vi "探头窗口-28-4列.vi"() -> ()   [LabVIEW 2017]
panel:
  in  "更新数据":T1
  in  "停止信号":bool=TRUE
  out "更新数据？":bool=TRUE
  out "引用-切回列表模式？":refnum<vi>
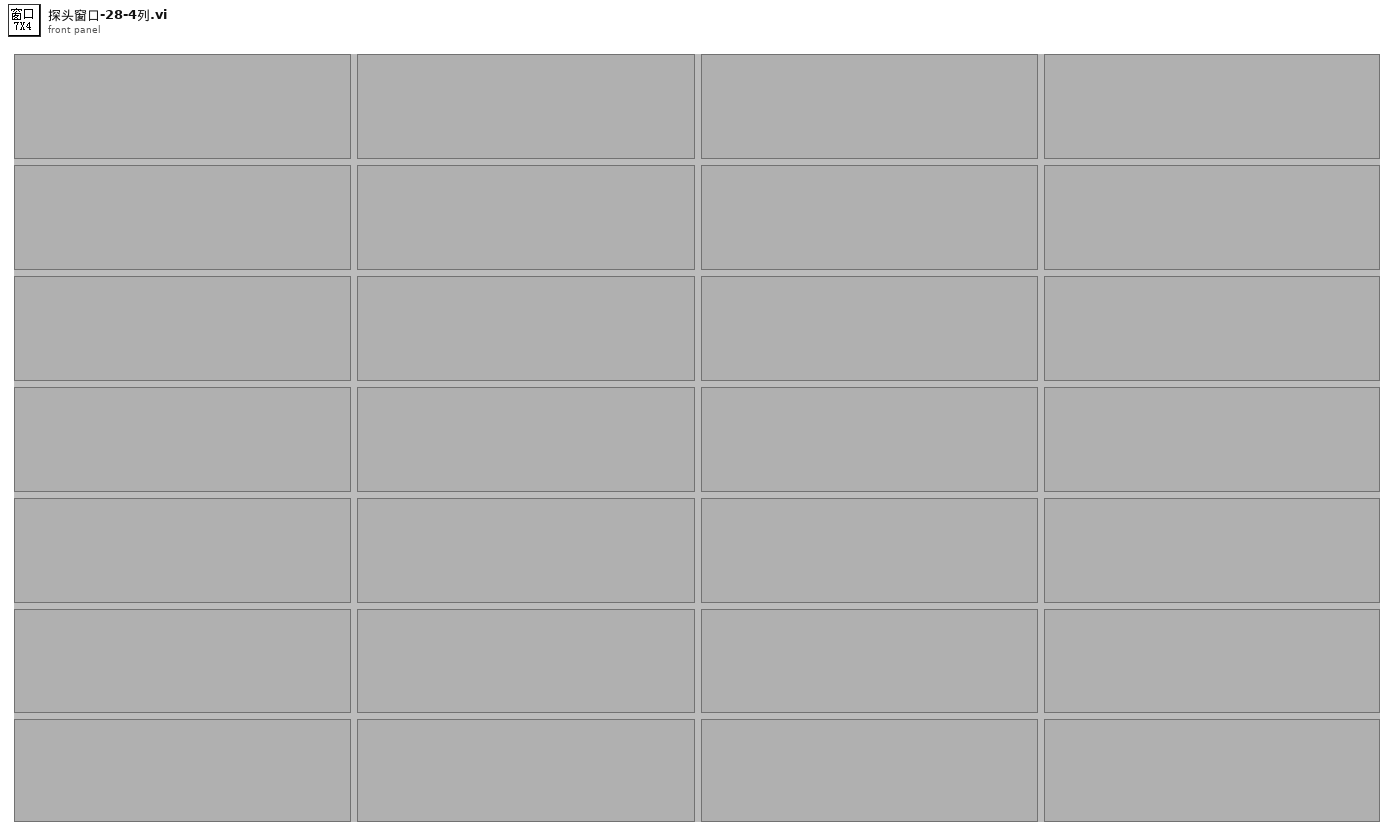
[diagram p1: front panel]
types:
  T1 = cluster{"探头启用状态？":bool[], "测量值":cluster{"X":timestamp, "Y":dbl}[], "限值":cluster{"限值1":dbl, "限值2":dbl, "探头限值":enum16{"一级限值", "二级限值"}}[], "报警状态":enum16{"正常", "一级报警", "二级报警", "累积报警"}[], "探头信息":string[], "累积剂量":cluster{"设备名称":string, "启用累积？":bool, "起始时间":timestamp, "累积剂量":dbl, "累积报警阈值":dbl}[]}
  T2 = cluster{"启用状态？":bool, "测量值":cluster{"X":timestamp, "Y":dbl}, "限值簇":cluster{"限值1":dbl, "限值2":dbl, "探头限值":enum16{"一级限值", "二级限值"}}, "报警状态":enum16{"正常", "一级报警", "二级报警", "累积报警"}, "探头信息":string, "探头地址":i32, "累积剂量":cluster{"设备名称":string, "启用累积？":bool, "起始时间":timestamp, "累积剂量":dbl, "累积报警阈值":dbl}}
  T3 = typedef "eventvkey.ctl" = enum16{"ASCII", "Enter", "Return", "Shift", "Ctrl", "Alt", "Cmd", "Opt", "Caps", "NumLock", "Clear", "Break", "Up", "Down", "Left", "Right", "Insert", "Delete", "Home", "End", "PageUp", "PageDown", "Escape", "Help", "Pause", "ScrollLock", "F1", "F2", "F3", "F4", "F5", "F6", "F7", "F8", "F9", "F10", "F11", "F12", "F13", "F14", "F15", "F16", "F17", "F18", "F19", "F20", "F21", "F22", "F23", "F24", "Play", "VolumeUp", "VolumeDown", "Mute", "Two Byte Char"}
  T4 = cluster{"限值1":dbl, "限值2":dbl, "探头限值":enum16{"一级限值", "二级限值"}}
  T5 = cluster{"限值1":dbl, "限值2":dbl, "探头限值":enum16{"一级限值", "二级限值"}}[]
  T6 = cluster{"设备名称":string, "启用累积？":bool, "起始时间":timestamp, "累积剂量":dbl, "累积报警阈值":dbl}[]
  T7 = cluster{"设备名称":string, "启用累积？":bool, "起始时间":timestamp, "累积剂量":dbl, "累积报警阈值":dbl}
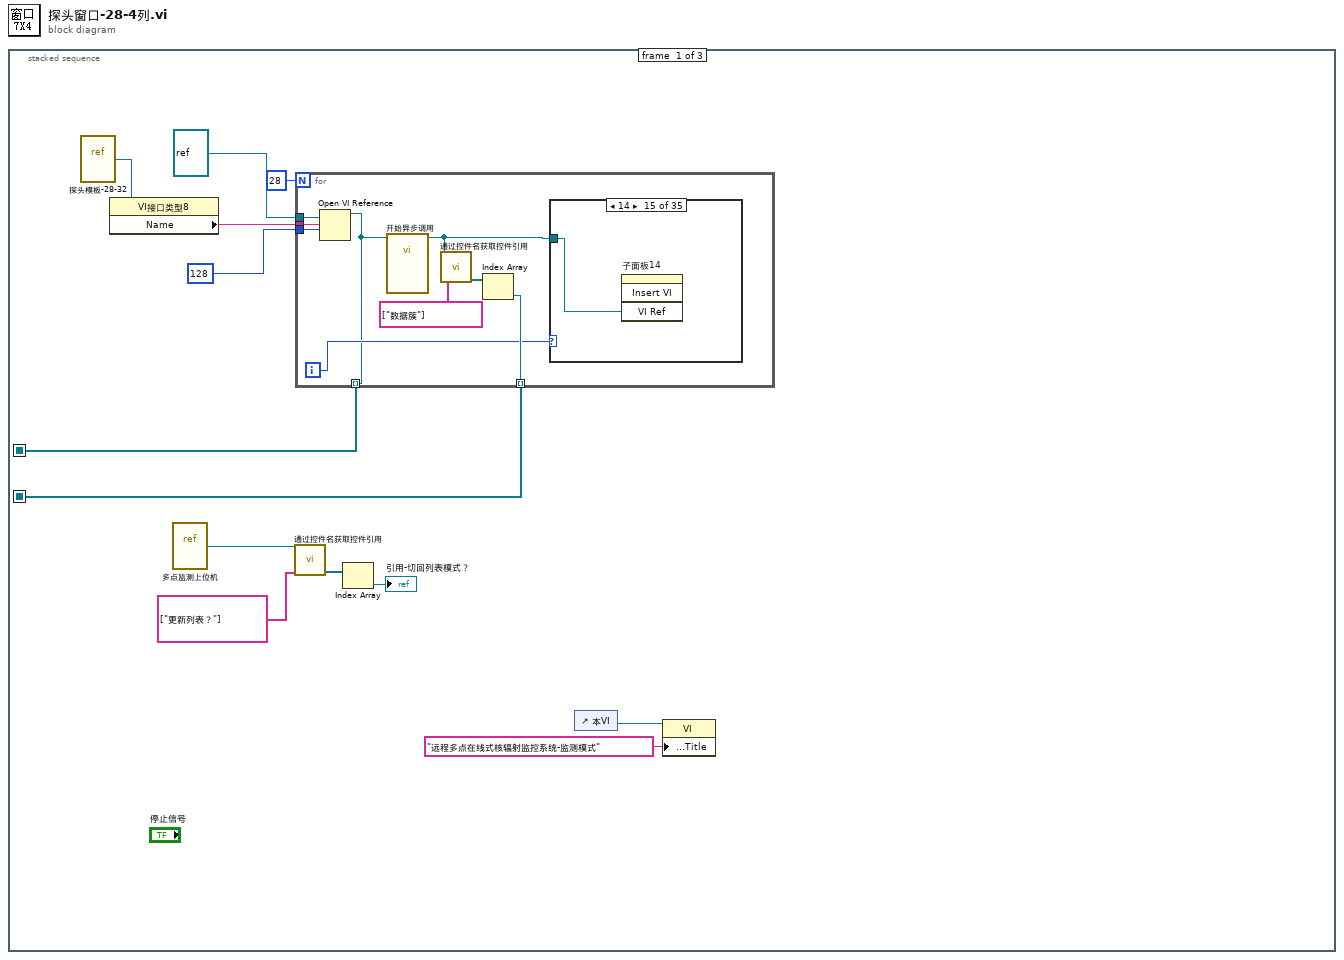
[diagram p0: block diagram]
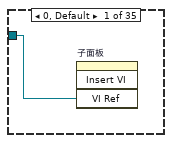
[diagram p2: hidden frame]
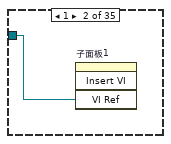
[diagram p3: hidden frame]
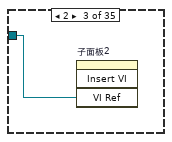
[diagram p4: hidden frame]
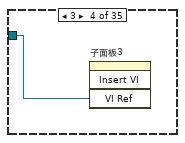
[diagram p5: hidden frame]
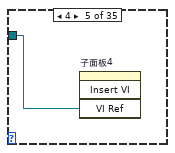
[diagram p6: hidden frame]
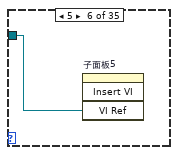
[diagram p7: hidden frame]
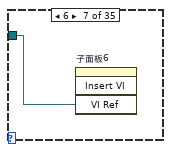
[diagram p8: hidden frame]
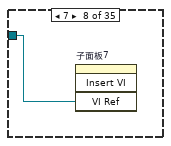
[diagram p9: hidden frame]
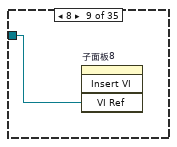
[diagram p10: hidden frame]
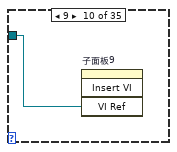
[diagram p11: hidden frame]
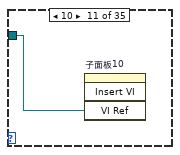
[diagram p12: hidden frame]
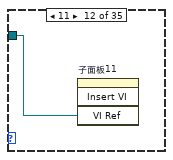
[diagram p13: hidden frame]
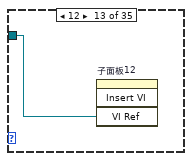
[diagram p14: hidden frame]
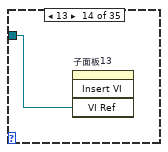
[diagram p15: hidden frame]
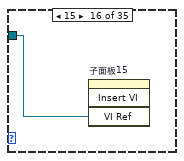
[diagram p16: hidden frame]
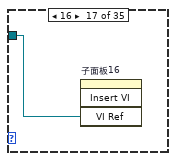
[diagram p17: hidden frame]
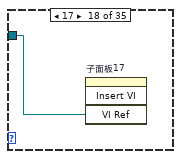
[diagram p18: hidden frame]
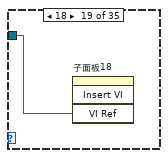
[diagram p19: hidden frame]
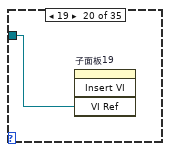
[diagram p20: hidden frame]
diagram:
  n1 = stacked-sequence {
    seq-local: [w8 _ _] -> [_ w52 _]
    seq-local: [w3 _ _] -> [_ w51 _]
    frame #0 {
      n2 = vi-ref "探头模板-28-32.vi"() -> (w13:refnum<vi>)
      n3 = property class="VI接口类型8"(reference=w13) -> ("Name"=w12:string)  [unwired: 1 in, 2 out]
      n4 = vi-ref "多点监测上位机.vi"() -> (w4:refnum<vi>)
      n5 = call "通过控件名获取控件引用.vi"("控件名数组"=string[] ["更新列表？"], "VI引用"=w4) -> ("控件引用输出"=w6:refnum<vi>[])  [unwired: 7 in, 2 out]
      n6 = for {
        N: 28 -> [_]
        tunnel: w12 -> [w22]
        tunnel: 128 ("选项") -> [w21]
        tunnel: refnum<vi> refnum ("类型说明符VI引用句柄（仅用于类型）") -> [w20]
        tunnel: [w15] -> w8 mode=indexing
        tunnel: [w17] -> w3 mode=indexing
        i -> [w16]
        n7 = Open VI Reference(type specifier VI Refnum (for type only)=w20, vi path=w22, options=w21) -> (vi reference=w15:refnum<vi>)  [unwired: 3 in, 1 out]
        n8 = call-by-ref "开始异步调用"(reference=w15) -> (reference out=w14:refnum<vi>)  [unwired: 13 in, 1 out]
        n9 = call "通过控件名获取控件引用.vi"("控件名数组"=string[] ["数据簇"], "VI引用"=w14) -> ("控件引用输出"=w19:refnum<vi>[])  [unwired: 7 in, 2 out]
        n10 = Index Array(array=w19) -> (element=w17:refnum<vi>)  [unwired: 1 in]
        n11 = case shown="14" w16 {
          tunnel: w14 -> [w23 w24 w25 w26 w27 w28 w29 w30 w31 w32 w33 w34 w35 w36 w37 w38 w39 w40 w41 w42 w43 w44 w45 w46 w47 w48 w49 w50 _ _ _ _ _ _ _]
          frame 0, Default {
            n12 = invoke on="子面板" class="子面板" method="Insert VI"("VI Ref"=w23) -> ()  [unwired: 3 in, 4 out]
          }
          frame 1 {
            n13 = invoke on="子面板1" class="SubPnl" method="Insert VI"("VI Ref"=w24) -> ()  [unwired: 3 in, 4 out]
          }
          frame 2 {
            n14 = invoke on="子面板2" class="SubPnl" method="Insert VI"("VI Ref"=w25) -> ()  [unwired: 3 in, 4 out]
          }
          frame 3 {
            n15 = invoke on="子面板3" class="SubPnl" method="Insert VI"("VI Ref"=w26) -> ()  [unwired: 3 in, 4 out]
          }
          frame 4 {
            n16 = invoke on="子面板4" class="SubPnl" method="Insert VI"("VI Ref"=w27) -> ()  [unwired: 3 in, 4 out]
          }
          frame 5 {
            n17 = invoke on="子面板5" class="SubPnl" method="Insert VI"("VI Ref"=w28) -> ()  [unwired: 3 in, 4 out]
          }
          frame 6 {
            n18 = invoke on="子面板6" class="SubPnl" method="Insert VI"("VI Ref"=w29) -> ()  [unwired: 3 in, 4 out]
          }
          frame 7 {
            n19 = invoke on="子面板7" class="SubPnl" method="Insert VI"("VI Ref"=w30) -> ()  [unwired: 3 in, 4 out]
          }
          frame 8 {
            n20 = invoke on="子面板8" class="SubPnl" method="Insert VI"("VI Ref"=w31) -> ()  [unwired: 3 in, 4 out]
          }
          frame 9 {
            n21 = invoke on="子面板9" class="SubPnl" method="Insert VI"("VI Ref"=w32) -> ()  [unwired: 3 in, 4 out]
          }
          frame 10 {
            n22 = invoke on="子面板10" class="SubPnl" method="Insert VI"("VI Ref"=w33) -> ()  [unwired: 3 in, 4 out]
          }
          frame 11 {
            n23 = invoke on="子面板11" class="SubPnl" method="Insert VI"("VI Ref"=w34) -> ()  [unwired: 3 in, 4 out]
          }
          frame 12 {
            n24 = invoke on="子面板12" class="SubPnl" method="Insert VI"("VI Ref"=w35) -> ()  [unwired: 3 in, 4 out]
          }
          frame 13 {
            n25 = invoke on="子面板13" class="SubPnl" method="Insert VI"("VI Ref"=w36) -> ()  [unwired: 3 in, 4 out]
          }
          frame 14 {
            n26 = invoke on="子面板14" class="SubPnl" method="Insert VI"("VI Ref"=w37) -> ()  [unwired: 3 in, 4 out]
          }
          frame 15 {
            n27 = invoke on="子面板15" class="SubPnl" method="Insert VI"("VI Ref"=w38) -> ()  [unwired: 3 in, 4 out]
          }
          frame 16 {
            n28 = invoke on="子面板16" class="SubPnl" method="Insert VI"("VI Ref"=w39) -> ()  [unwired: 3 in, 4 out]
          }
          frame 17 {
            n29 = invoke on="子面板17" class="SubPnl" method="Insert VI"("VI Ref"=w40) -> ()  [unwired: 3 in, 4 out]
          }
          frame 18 {
            n30 = invoke on="子面板18" class="SubPnl" method="Insert VI"("VI Ref"=w41) -> ()  [unwired: 3 in, 4 out]
          }
          frame 19 {
            n31 = invoke on="子面板19" class="SubPnl" method="Insert VI"("VI Ref"=w42) -> ()  [unwired: 3 in, 4 out]
          }
          frame 20 {
            n32 = invoke on="子面板20" class="SubPnl" method="Insert VI"("VI Ref"=w43) -> ()  [unwired: 3 in, 4 out]
          }
          frame 21 {
            n33 = invoke on="子面板21" class="SubPnl" method="Insert VI"("VI Ref"=w44) -> ()  [unwired: 3 in, 4 out]
          }
          frame 22 {
            n34 = invoke on="子面板22" class="SubPnl" method="Insert VI"("VI Ref"=w45) -> ()  [unwired: 3 in, 4 out]
          }
          frame 23 {
            n35 = invoke on="子面板23" class="SubPnl" method="Insert VI"("VI Ref"=w46) -> ()  [unwired: 3 in, 4 out]
          }
          frame 24 {
            n36 = invoke on="子面板24" class="SubPnl" method="Insert VI"("VI Ref"=w47) -> ()  [unwired: 3 in, 4 out]
          }
          frame 25 {
            n37 = invoke on="子面板25" class="SubPnl" method="Insert VI"("VI Ref"=w48) -> ()  [unwired: 3 in, 4 out]
          }
          frame 26 {
            n38 = invoke on="子面板26" class="SubPnl" method="Insert VI"("VI Ref"=w49) -> ()  [unwired: 3 in, 4 out]
          }
          frame 27 {
            n39 = invoke on="子面板27" class="SubPnl" method="Insert VI"("VI Ref"=w50) -> ()  [unwired: 3 in, 4 out]
          }
          frame 28 {
          }
          frame 29 {
          }
          frame 30 {
          }
          frame 31 {
          }
          frame 32 {
          }
          frame 33 {
          }
          frame 34 {
          }
        }
      }
      n40 = Index Array(array=w6) -> (element=→"引用-切回列表模式？":refnum<vi>)  [unwired: 1 in]
      n41 = control-ref of="本VI"() -> (w2:refnum<vi>)
      n42 = property class="VI"(reference=w2, "Front Panel.Title"="远程多点在线式核辐射监控系统-监测模式" ("前面板窗口:标题")) -> ()  [unwired: 1 in, 2 out]
    }
    frame #1 {
      n43 = while {
        tunnel: w52 -> [w54]
        tunnel: w51 -> [w53]
        stop <- w55 stop-if-true
        n44 = event shown="[4] \"更新数据？\": 值改变" {
          selector: _ -> [_ _ _ _ _]
          dyn-events: _ -> [_ _ _ _ _]
          timeout: _ -> [_ _ _ _ _]
          tunnel: [_ TRUE ("放弃？") _ _ _] -> w55
          tunnel: w54 -> [_ w58 _ _ _]
          tunnel: w53 -> [_ _ _ _ w67]
          event Timeout {
            n45 = event-data() -> ()  [unwired: 1 in, 3 out]
          }
          event "停止信号": Value Change {
            w57 = TRUE  # T
            n46 = event-data() -> ()  [unwired: 1 in, 6 out]
            n47 = local read "引用-切回列表模式？"() -> (w56:refnum<vi>)
            n48 = for {
              tunnel: w58 -> [w63] mode=indexing
              n49 = invoke class="VI (严格)" method="Abort VI"(reference=w63) -> (reference out=w61:refnum<vi>, error out=w62:errorcluster)  [unwired: 2 in, 1 out]
              n50 = Close Reference(reference=w61, error in (no error)=w62) -> (error out=w60:errorcluster)
              n51 = call <vilib>:"Clear Errors.vi"("error in (no error)"=w60) -> ()  [unwired: 5 in, 2 out]
            }
            n52 = property class="Ctl"(reference=w56, "Val(Sgnl)"=w57) -> ()  [unwired: 1 in, 2 out]
          }
          event Panel Close? {
            n53 = event-data() -> ()  [unwired: 1 in, 4 out]
            n54 = property on="停止信号" class="Bool (严格)"("Val(Sgnl)"=FALSE ("值(信号)")) -> ()  [unwired: 2 in, 2 out]
            n55 = event-data() -> ()  [unwired: 2 in, 1 out]
          }
          event Key Down {
            n56 = event-data() -> ("VKey"=w65:T3)  [unwired: 1 in, 9 out]
            n57 = case shown="\"Escape\"" w65 {
              frame "ASCII", Default {
              }
              frame "Escape" {
                w66 = TRUE  # T
                n58 = property on="停止信号" class="Bool (严格)"("Val(Sgnl)"=w66) -> ()  [unwired: 2 in, 2 out]
              }
            }
          }
          event "更新数据？": Value Change {
            (unwired) T4 {"限值1"=0.0, "限值2"=0.0, "探头限值"=enum."一级限值"} ("探头限值簇")
            n59 = event-data() -> ()  [unwired: 1 in, 6 out]
            n60 = Unbundle By Name("更新数据") -> ("探头启用状态？"=w68:bool[], "测量值"=w69:cluster{"X":timestamp, "Y":dbl}[], "限值"=w70:T5, "报警状态"=w71:enum16{"正常", "一级报警", "二级报警", "累积报警"}[], "探头信息"=w72:string[], "累积剂量"=w73:T6)
            n61 = for {
              tunnel: w68 -> [w87] mode=indexing
              tunnel: w69 -> [w86] mode=indexing
              tunnel: w70 -> [w85] mode=indexing
              tunnel: w71 -> [w84] mode=indexing
              tunnel: w72 -> [w79] mode=indexing
              workers-P: _ -> [_]
              tunnel: w67 -> [w82] mode=indexing
              tunnel: w73 -> [w78]
              i -> [w80]
              # "分配出 各个探头的数据簇，然后赋值"
              n62 = for {
                tunnel: w78 -> [w97] mode=indexing
                tunnel: w79 -> [w95]
                tunnel: [w92] -> w77
                tunnel: [w91] -> w76
                i -> [w92]
                stop <- w91 stop-if-true
                # "查找匹配，获取索引"
                n63 = Unbundle By Name(w97) -> ("设备名称"=w96:string, "启用累积？"=w93:bool)
                n64 = Equal? "匹配？"(x=w95, y=w96) -> (x = y?=w94:bool)
                n65 = And(x=w94, y=w93) -> (x .and. y?=w91:bool)
              }
              n66 = case shown="真" w76 {
                tunnel: w78 -> [_ w90]
                tunnel: w77 -> [_ w89]
                tunnel: [_ w88] -> w75
                frame False {
                  # "不匹配"
                }
                frame True {
                  # "匹配"
                  n67 = Index Array(array=w90, index=w89) -> (element=w88:T7)
                }
              }
              n68 = Bundle By Name(cluster=T2 {"启用状态？"=FALSE, "测量值"={"X"=timestamp(0 s since 1904-01-01), "Y"=0.0}, "限值簇"={"限值1"=0.0, "限值2"=0.0, "探头限值"=enum."一级限值"}, "报警状态"=enum."正常", "探头信息"="", "探头地址"=0, "累积剂量"={"设备名称"="", "启用累积？"=FALSE, "起始时间"=timestamp(0 s since 1904-01-01), "累积剂量"=0.0, "累积报警阈值"=0.0}} ("输出簇"), "启用状态？"=w87, "测量值"=w86, "限值簇"=w85, "报警状态"=w84, "探头信息"=w79, "探头地址"=w80, "累积剂量"=w75) -> (w81:T2)
              n69 = property class="Ctl"(reference=w82, "Val(Sgnl)"=w81) -> ()  [unwired: 1 in, 2 out]
            }
          }
        }
      }
    }
    frame #2 {
      n70 = control-ref of="本VI"() -> (w101:refnum<vi>)
      n71 = invoke class="VI" method="FP.Close"(reference=w101) -> (reference out=w100:refnum<vi>, error out=w99:errorcluster)  [unwired: 2 in, 1 out]
      n72 = invoke class="VI" method="Abort VI"(reference=w100, error in=w99) -> (error out=w98:errorcluster)  [unwired: 1 in, 2 out]
      n73 = call <vilib>:"Clear Errors.vi"("error in (no error)"=w98) -> ()  [unwired: 5 in, 2 out]
    }
  }
